vi "TimeInterpBoolean_CleanUp.vi"(11 "in TimeInterpBoolean":T1) -> (0 "Error":bool, 3 "out TimeInterpBoolean":T1)   [LabVIEW 2019, in "Trajectory_Library.lvlib"]
doc: "Removes samples older than our current history size.\n\nInputs:\n - In TimeInterpBoolean -- Input data cluster.\n\nOutputs:\n - Out TimeInterpBoolean -- Updated data cluster.\n - Error -- Returns TRUE if an error occured."
uses:
  Trajectory_Library.lvlib
  TypeDef/TIME_INTERPOLATABLE_BOOLEAN.ctl
  <vilib>/gmath/NI_Gmath.lvlib
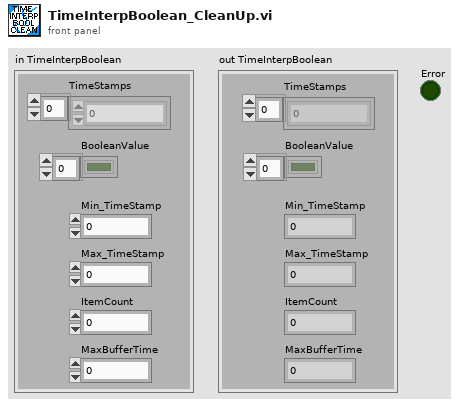
[diagram p1: front panel]
types:
  T1 = typedef "Trajectory_Library.lvlib/TIME_INTERPOLATABLE_BOOLEAN.ctl" = cluster{"TimeStamps":dbl[], "BooleanValue":bool[], "Min_TimeStamp":dbl, "Max_TimeStamp":dbl, "ItemCount":i32, "MaxBufferTime":dbl}
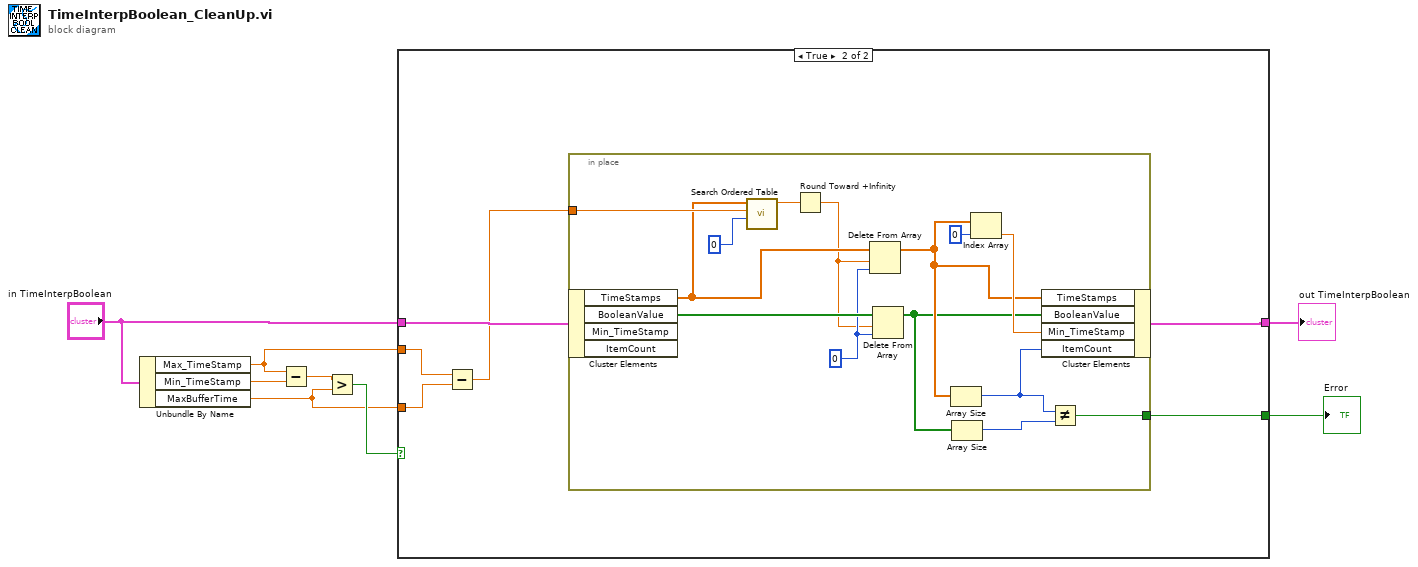
[diagram p0: block diagram]
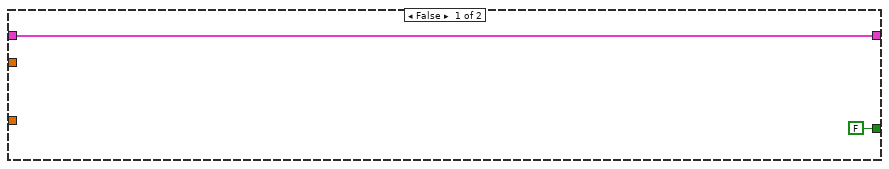
[diagram p2: hidden frame]
diagram:
  n1 = Unbundle By Name("in TimeInterpBoolean") -> ("Max_TimeStamp"=w3:dbl, "Min_TimeStamp"=w6:dbl, "MaxBufferTime"=w2:dbl)
  n2 = Subtract(x=w3, y=w6) -> (x-y=w5:dbl)
  n3 = Greater?(x=w5, y=w2) -> (0:w4:bool)
  n4 = case shown="True" w4 {
    tunnel: "in TimeInterpBoolean" -> [w10 w14]
    tunnel: [w10 w12] -> w8
    tunnel: w3 -> [_ w16]
    tunnel: w2 -> [_ w15]
    tunnel: [FALSE w11] -> w1
    frame False {
    }
    frame True {
      n5 = Subtract(x=w16, y=w15) -> (x-y=w13:dbl)
      n6 = in-place {
        in-place-border: w13 -> [w29]
        in-place-border: [w17] -> w11
        w25 = 0 ("index")
        n7 = in-place-cluster #1(w14) -> ("TimeStamps"=w28:dbl[], "BooleanValue"=w27:bool[])  [unwired: 2 out]
        n8 = call <vilib>:"Search Ordered Table.vi"("starting index"=0, "x value"=w29, "ordered x array"=w28) -> ("fractional index"=w26:dbl)  [unwired: 8 in]
        n9 = Round Toward +Infinity(x=w26) -> (ceil(x): smallest int >= x=w24:dbl)
        n10 = Delete From Array(array=w28, length=w24, index=w25) -> (array with subset deleted=w21:dbl[])  [unwired: 1 out]
        n11 = Delete From Array(array=w27, length=w24, index=w25) -> (array with subset deleted=w20:bool[])  [unwired: 1 out]
        n12 = Array Size(array=w21) -> (size(s)=w19:i32)
        n13 = Array Size(array=w20) -> (size(s)=w18:i32)
        n14 = Index Array(array=w21, index=0) -> (element=w22:dbl)
        n15 = in-place-cluster #1("TimeStamps"=w21, "BooleanValue"=w20, "Min_TimeStamp"=w22, "ItemCount"=w19) -> (w12:T1)
        n16 = Not Equal?(x=w19, y=w18) -> (x != y?=w17:bool)
      }
    }
  }
  "out TimeInterpBoolean" <- w8
  "Error" <- w1
